vi "tio32_Close.vi"(5 "error in (no error)":errorcluster, 8 "VISA resource name":refnum<visa-resource-name>) -> (0 "error out":errorcluster, 2 "return":i32=666, 3 "VISA resource name out":refnum<visa-resource-name>)   [LabVIEW 2011]
doc: "DLL tio32.dll\nFunction INT16TYPE WINAPI tio32_Close(void);\n\nClose the DLL."
uses:
  l_pse_dll/Tio32.dll
panel:
  # "tio32_Close"
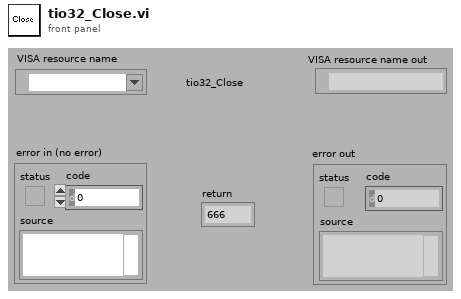
[diagram p1: front panel]
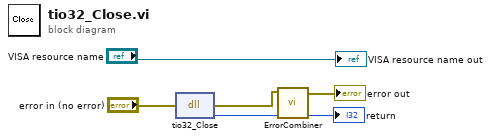
[diagram p0: block diagram]
diagram:
  n1 = dll-call lib="C:/Users/Ikaika's/Documents/DCC/Apps/INA231/INA231-SFT-rev1/INA231-Sourcecode-rev1/INA231/Shell Resources/l_pse_dll/Tio32.dll" fn="tio32_Close"(error in="error in (no error)") -> (error out=w2:errorcluster, "Rückgabetyp"=w1:i32)  [unwired: 2 in, 1 out]
  n2 = call "ErrorCombiner.vi"("Return In"=w1, "error in (no error)"=w2) -> ("Return Out"=→"return":i32, "error out"=→"error out":errorcluster)  [unwired: 8 in]
  "VISA resource name out" <- "VISA resource name"
